vi "FlatToRichrfcontrol_TemperatureReadings.vi"(5 "OutputClusterType":T1, 11 "InputCluster":T2) -> (3 "OutputCluster":T1)   [LabVIEW 2024, in "FlexSDR_gRPC_client.lvlib"]
uses:
  FlexSDR_gRPC_client.lvlib
  rfcontrol_TemperatureReadings_Flat.ctl
  rfcontrol_TemperatureReadings.ctl
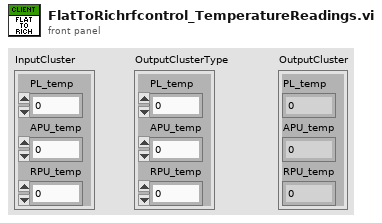
[diagram p1: front panel]
types:
  T1 = typedef "FlexSDR_gRPC_client.lvlib/rfcontrol_TemperatureReadings.ctl" = cluster{"PL_temp":dbl, "APU_temp":dbl, "RPU_temp":dbl}
  T2 = typedef "FlexSDR_gRPC_client.lvlib/rfcontrol_TemperatureReadings_Flat.ctl" = cluster{"PL_temp":dbl, "APU_temp":dbl, "RPU_temp":dbl}
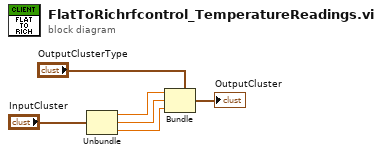
[diagram p0: block diagram]
diagram:
  n1 = Unbundle "Unbundle"("InputCluster") -> ("PL_temp"=w3:dbl, "APU_temp"=w2:dbl, "RPU_temp"=w1:dbl)
  n2 = Bundle "Bundle"(cluster="OutputClusterType", "PL_temp"=w3, "APU_temp"=w2, "RPU_temp"=w1) -> (→"OutputCluster":T1)
